vi "emi_BCD U8 to Num U8.vi"(7 "BCD":u8) -> (8 "Numeric":u8, 10 "Valid Numeric BCD":bool)   [LabVIEW 2010]
doc: "BCD must keep have a bcd coded value between 0 and 99. Lo Nibble must be 0 - 9, Hi Nibble must be 0-9. If either nibble is higher, A-F, Numeric will not be a valid number and \"Valid Numeric BCD\" will be False.\n\nResult will be a hex value with value between 0 and 99 (if valid)."
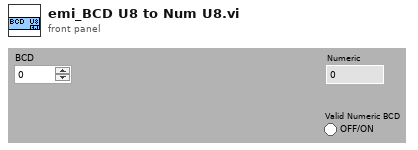
[diagram p1: front panel]
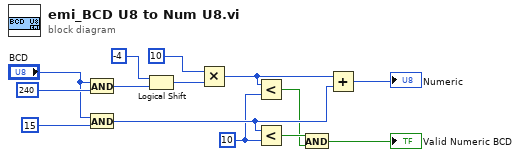
[diagram p0: block diagram]
diagram:
  w4 = u8 10 ("y")
  n1 = And(x="BCD", y=u8 240) -> (x .and. y?=w13:u8)
  n2 = And(x="BCD", y=u8 15) -> (x .and. y?=w5:u8)
  n3 = Logical Shift(y=i8 -4, x=w13) -> (x << y=w9:u8)
  n4 = Multiply(x=u8 10, y=w9) -> (x*y=w6:u8)
  n5 = Less?(x=w6, y=w4) -> (x < y?=w2:bool)
  n6 = Less?(x=w5, y=w4) -> (x < y?=w3:bool)
  n7 = And(x=w3, y=w2) -> (x .and. y?=→"Valid Numeric BCD":bool)
  n8 = Add(x=w6, y=w5) -> (x+y=→"Numeric":u8)
